vi "Save Chunk.vi"(8 "error in (no error)":errorcluster, 9 "Voltage":cdb[](array[numeric]), 10 "Frequency":dbl[](array[numeric]), 11 "Spectrum Recorder in":refnum<class "Spectrum Recorder.lvclass">) -> (0 "error out":errorcluster, 3 "Spectrum Recorder out":refnum<class "Spectrum Recorder.lvclass">)   [LabVIEW 2016, in "Spectrum Recorder.lvclass"]
uses:
  Spectrum Recorder.lvclass
  Spectrum Recorder.lvclass/Spectrum Recorder.ctl
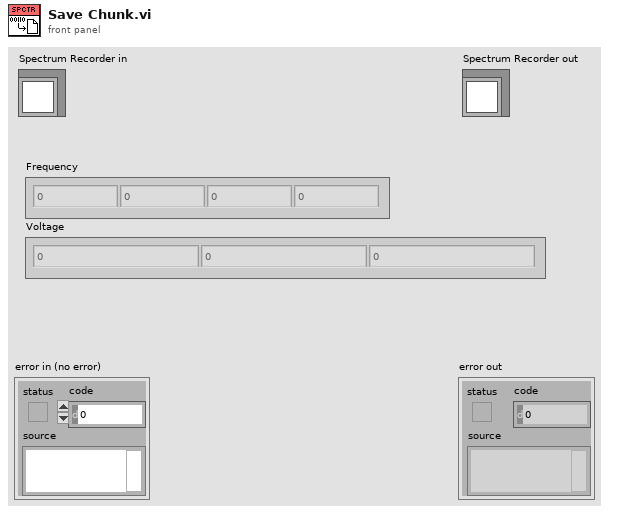
[diagram p1: front panel]
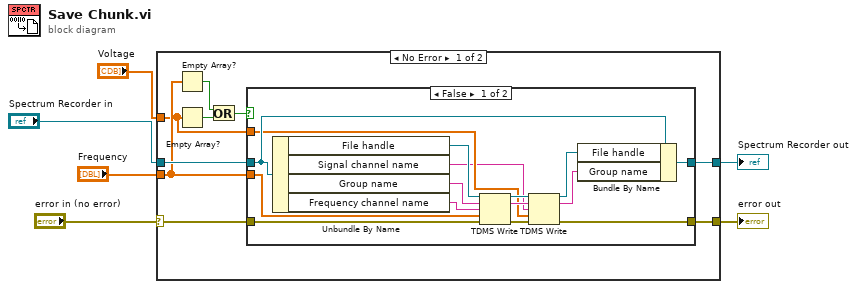
[diagram p0: block diagram]
diagram:
  n1 = case shown="No Error" "error in (no error)" {
    selector: "error in (no error)" -> [w13 w34]
    tunnel: [w12 w34] -> w5
    tunnel: [w14 w33] -> w3
    tunnel: "Spectrum Recorder in" -> [w15 w33]
    tunnel: "Voltage" -> [w7 _]
    tunnel: "Frequency" -> [w8 _]
    frame No Error {
      n2 = Empty Array?(array=w8) -> (empty?=w11:bool)
      n3 = Empty Array?(array=w7) -> (empty?=w10:bool)
      n4 = Or(x=w11, y=w10) -> (x .or. y?=w9:bool)
      n5 = case shown="False" w9 {
        tunnel: w7 -> [w19 _]
        tunnel: w8 -> [w25 _]
        tunnel: w15 -> [w28 w32]
        tunnel: [w27 w32] -> w14
        tunnel: w13 -> [w26 w31]
        tunnel: [w18 w31] -> w12
        frame False {
          n6 = Unbundle By Name(w28) -> ("File handle"=w30:refnum<k34>, "Signal channel name"=w16:string, "Group name"=w29:string, "Frequency channel name"=w17:string)
          n7 = TDMS Write(0:w30, 5:w29, 7:w17, 9:w25, 11:w26) -> (4:w22:refnum<k34>, 6:w21:string, 15:w24:errorcluster)  [unwired: 1 in, 1 out]
          n8 = TDMS Write(0:w22, 5:w21, 7:w16, 9:w19, 11:w24) -> (4:w23:refnum<k34>, 6:w20:string, 15:w18:errorcluster)  [unwired: 1 in, 1 out]
          n9 = Bundle By Name(cluster=w28, "File handle"=w23, "Group name"=w20) -> (w27:refnum<class "Spectrum Recorder.lvclass">)
        }
        frame True {
        }
      }
    }
    frame Error {
    }
  }
  "error out" <- w5
  "Spectrum Recorder out" <- w3
